vi "Keithley Sweep_IIT.vi"(5 "Sweep Direction":u16(ring) items=["Low to high", "High to low"], 6 "Number of Points":u32=5, 7 "Maximum Amplitude":dbl=2.0, 8 "Minimum Amplitude":dbl=1.0, 9 "VISA resource name out 2":refnum<visa-resource-name>) -> (0 "Measurement Complete":bool, 2 "Data Array":dbl[][](array[numeric]), 3 "VISA resource name out":refnum<visa-resource-name>)   [LabVIEW 2011]
doc: "Configures a sweep and takes voltage and current readings at each point."
uses:
  <instrlib>/keithley_24xx/Keithley 24XX/Public/Data/Read (Multiple Points).vi
  <instrlib>/keithley_24xx/Keithley 24XX/Keithley 24XX.lvlib
panel:
  in  "Source Mode  (0: Voltage)":u16(ring) items=["Voltage", "Current"]
  # "(c) 2006 National Instruments.  ALL RIGHTS RESERVED."
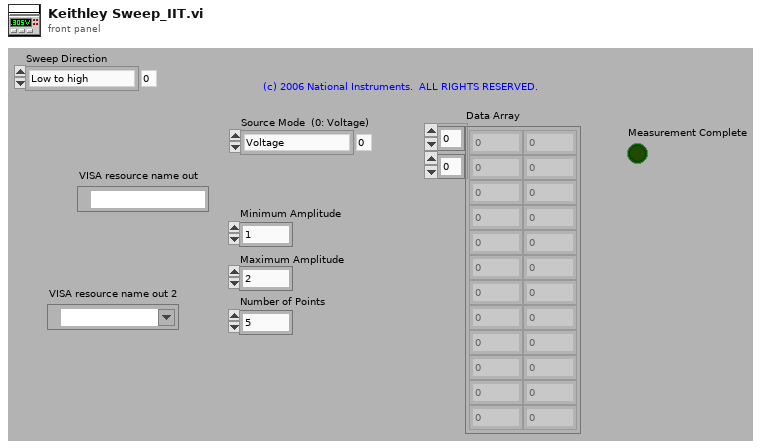
[diagram p1: front panel]
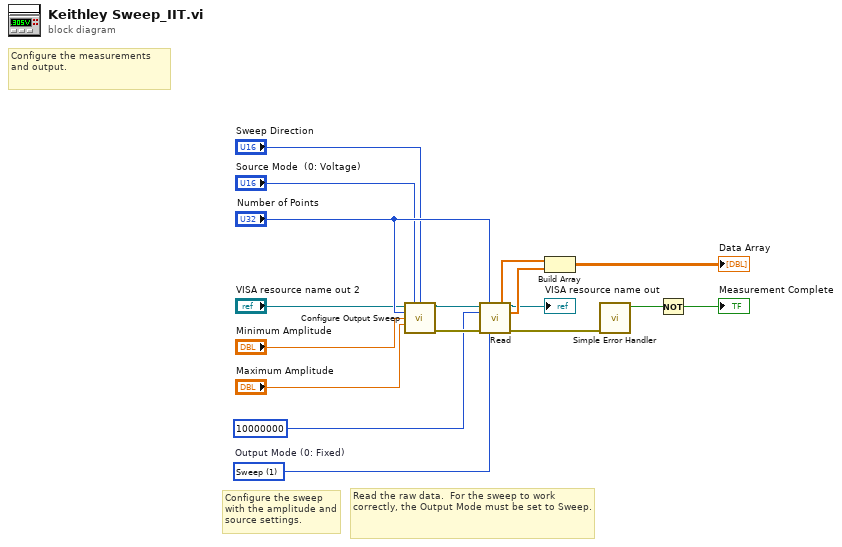
[diagram p0: block diagram]
diagram:
  w12 = u16 1 items=["Fixed", "Sweep", "List"]  # Output Mode (0: Fixed)
  # "Read the raw data.  For the sweep to work correctly, the Output Mode must be set to Sweep."
  # "Configure the sweep with the amplitude and source settings."
  # "Configure the measurements and output."
  n1 = call <instrlib>:"Configure Output Sweep.vi"("VISA resource name"="VISA resource name out 2", "Source Mode  (0: Voltage)"="Source Mode  (0: Voltage)", "Sweep Direction  (0: Ascending)"="Sweep Direction", "Number of Points (5)"="Number of Points", "Minimum Amplitude (1)"="Minimum Amplitude", "Maximum Amplitude (2)"="Maximum Amplitude") -> ("VISA resource name out"=w3:refnum<visa-resource-name>, "error out"=w2:errorcluster)  [unwired: 8 in]
  n2 = call-poly <instrlib>:"Read.vi"("VISA resource name"=w3, "Sample Count (1)"="Number of Points", "Timeout (10000 ms)"=10000000, "error in (no error)"=w2, "Output Mode (0: Fixed)"=w12) -> ("Voltage"=w15:sgl[], "VISA resource name out"=→"VISA resource name out":refnum<visa-resource-name>, "Current"=w14:sgl[], "error out"=w10:errorcluster)  [unwired: 4 in, 3 out]
  n3 = Build Array(w15, w14) -> (→"Data Array":sgl[][])
  n4 = call <vilib>:"Simple Error Handler.vi"("error in (no error)"=w10) -> ("error?"=w8:bool)  [unwired: 4 in, 4 out]
  n5 = Not(x=w8) -> (.not. x?=→"Measurement Complete":bool)
